vi "Get Mode.vi"(8 "error in (no error)":errorcluster, 11 "CnPt in":refnum<class "CnPt.lvclass">) -> (0 "error out":errorcluster, 2 "Mode":T1 items=["RUN"=6, "STANDBY"=7, "STOP"=8, "PAUSE"=9], 3 "CnPt out":refnum<class "CnPt.lvclass">)   [LabVIEW 2015, in "CnPt.lvclass"]
uses:
  CnPt.lvclass
  Mode.ctl
  <vilib>/MSR Consulting, LLC/General Reuse/Session APIs/Serial/Serial Session.lvclass
  CnPt.lvclass/CnPt.ctl
  <vilib>/MSR Consulting, LLC/General Reuse/Session APIs/Serial/Public/Asynchronous Write.vi
  <vilib>/MSR Consulting, LLC/General Reuse/Session APIs/Serial/Public/Asynchronous Read.vi
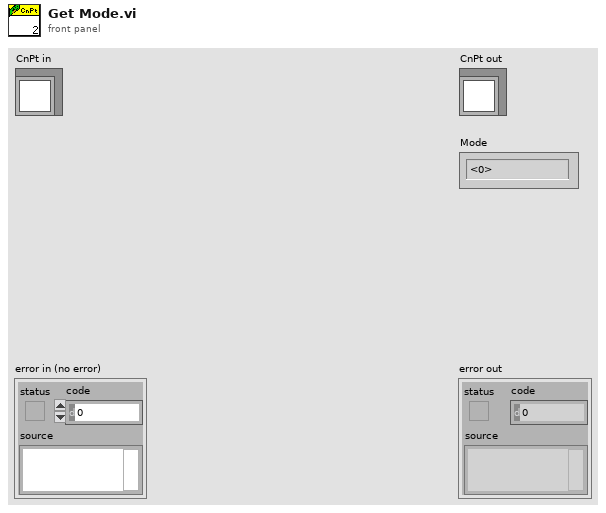
[diagram p1: front panel]
types:
  T1 = typedef "CnPt.lvclass/Mode.ctl" = u16
  T2 = typedef "Serial Session.lvclass/Session Handle.ctl" = refnum<data-value>
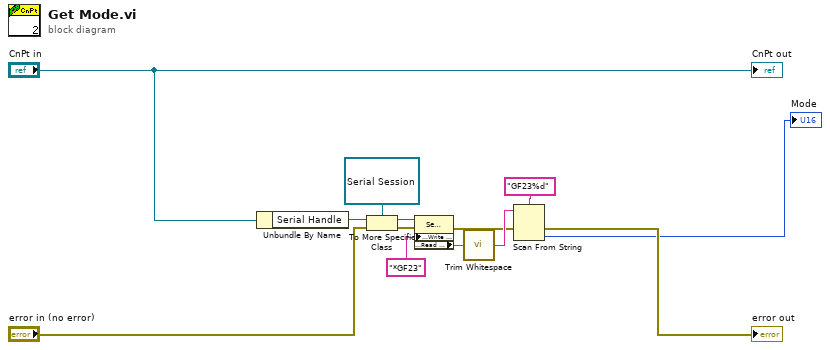
[diagram p0: block diagram]
diagram:
  n1 = Unbundle By Name("CnPt in") -> ("Serial Handle"=w13:T2)
  n2 = To More Specific Class(target class=refnum<data-value> refnum, reference=w13, error in="error in (no error)") -> (specific class reference=w11:refnum<data-value>, error out=w9:errorcluster)
  n3 = property class="Serial Session"(reference=w11, error in=w9, "Public:Write - Asynchronous"="*GF23" ("format string")) -> (error out=w5:errorcluster, "Public:Read - Asynchronous"=w7:string)  [unwired: 1 out]
  n4 = call <vilib>:"Trim Whitespace.vi"("string"=w7) -> ("trimmed string"=w6:string)  [unwired: 1 in]
  n5 = Scan From String(format string="GF23%d", input string=w6, error in=w5) -> (error out=→"error out":errorcluster, output 1=→"Mode":T1)  [unwired: 2 in, 2 out]
  "CnPt out" <- "CnPt in"
